vi "Manipulator Get Low Limit.vi"(8 "error in (no error)":errorcluster, 11 "VISA resource in":refnum<visa-resource-name>="COM1") -> (0 "error out":errorcluster, 2 "Low Limit":i32, 3 "VISA resource out":refnum<visa-resource-name>)   [LabVIEW 2012, in "Scientifica Manipulator Daemon.lvlib"]
uses:
  Scientifica Manipulator Daemon.lvlib
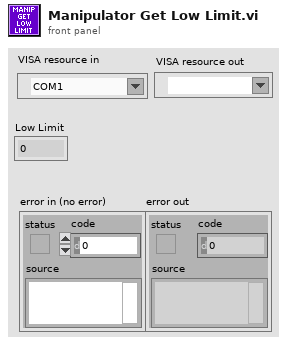
[diagram p1: front panel]
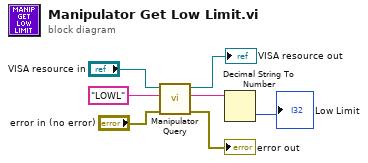
[diagram p0: block diagram]
diagram:
  n1 = call "Manipulator Query.vi"("error in (no error)"="error in (no error)", "Command"="LOWL", "VISA resource in"="VISA resource in") -> ("error out"=→"error out":errorcluster, "Response"=w2:string, "VISA resource out"=→"VISA resource out":refnum<visa-resource-name>)  [unwired: 5 in, 1 out]
  n2 = Decimal String To Number(string=w2) -> (number=→"Low Limit":i32)  [unwired: 2 in, 1 out]
